vi "19.6-DirectIIR-SinglePole-HP.vi"() -> ()   [LabVIEW 2020]
doc: "Uses the Median Filter VI to analyze pulses in the presence of noise. The example generates a pulse contaminated with Gaussian noise and applies a median filter. For comparison purposes, the VI computes the pulse parameters of the filtered pulse."
uses:
  <vilib>/Analysis/3filter.llb/IIR Filter (DBL).vi
  <vilib>/Analysis/NI_AALBase.lvlib
panel:
  in  "stop":bool
  out "H[k] 2":dbl[](graph)
  out "Filtered2":dbl[](graph)
  out "Filtered1":dbl[](graph)
  out "H[k]1":dbl[](graph)
  out "p":dbl format="%.2f"
  in  "Fc":dbl(slide)=25.974025974025974 scale=0.0..400.0
  in  "Fs":dbl(slide)=1024.0 scale=800.0..1024.0
  out "Sig":dbl[](graph)
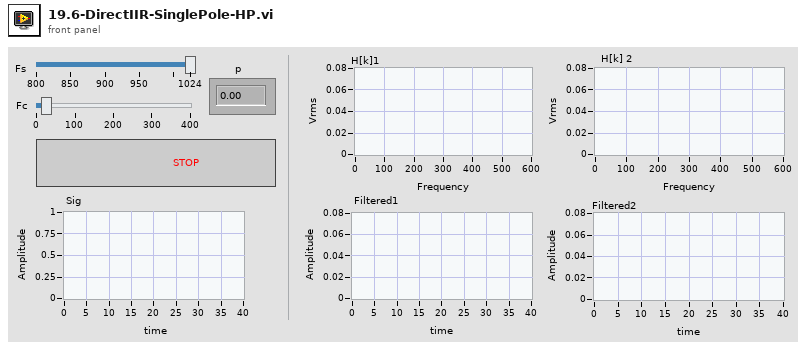
[diagram p1: front panel]
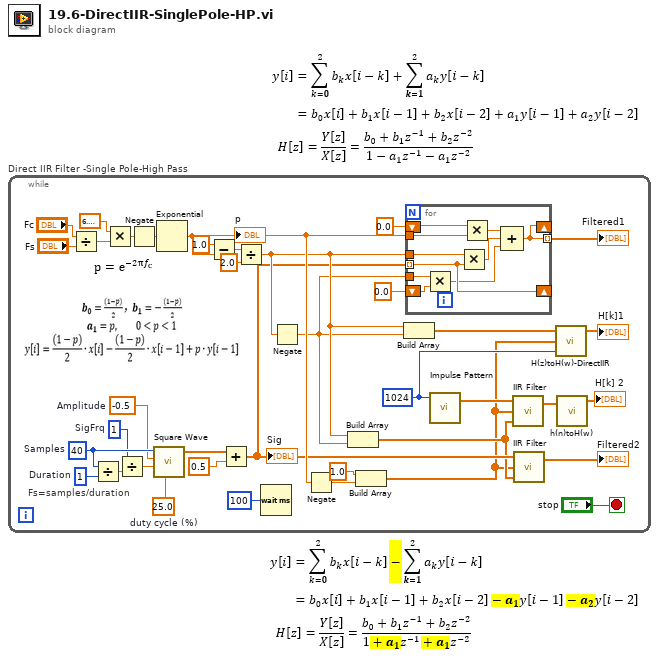
[diagram p0: block diagram]
diagram:
  n1 = while "Direct IIR Filter -Single Pole-High Pass" {
    stop <- "stop" stop-if-true
    w11 = 1  # Duration
    w8 = 1  # SigFrq
    w6 = 25.0  # duty cycle (%)
    w7 = -0.5  # Amplitude
    w10 = 40  # Samples
    w2 = 1024 ("samples")
    # "Fs=samples/duration"
    n2 = Divide(x="Fc", y="Fs") -> (x/y=w27:dbl)
    n3 = Divide(x=w10, y=w11) -> (x/y=w21:dbl)
    n4 = Multiply(x=6.283185307179586, y=w27) -> (x*y=w25:dbl)
    n5 = Divide(x=w8, y=w21) -> (x/y=w20:dbl)
    n6 = Negate(x=w25) -> (-x=w26:dbl)
    n7 = call <vilib>:"Square Wave.vi"("samples"=w10, "amplitude"=w7, "frequency"=w20, "duty cycle (%)"=w6) -> ("square wave"=w19:dbl[])  [unwired: 2 in, 2 out]
    n8 = Exponential(1:w26) -> (0:w31:dbl)
    "p" <- w31
    n9 = Subtract(x=1.0, y=w31) -> (x-y=w28:dbl)
    n10 = Add(x=w19, y=0.5) -> (x+y=w22:dbl[])
    "Sig" <- w22
    n11 = Divide(x=w28, y=2.0) -> (x/y=w30:dbl)
    n12 = Wait (ms)(milliseconds to wait=u32 100) -> ()  [unwired: 1 out]
    n13 = Negate(x=w30) -> (-x=w29:dbl)
    n14 = Negate(x=w31) -> (-x=w16:dbl)
    n15 = Build Array(w30, w29) -> (w17:dbl[])
    n16 = Build Array(1.0 ("element"), w16) -> (w1:dbl[])
    n17 = Build Array(w30, w29) -> (w15:dbl[])
    n18 = for {
      tunnel: w22 -> [w45] mode=indexing
      shift-right: [w39] -> _
      shift-left: 0.0 -> [w48]
      tunnel: w31 -> [w47]
      tunnel: w30 -> [w46]
      tunnel: [w39] -> w35 mode=indexing
      shift-right: [w45] -> _
      shift-left: 0.0 -> [w43]
      tunnel: w29 -> [w44]
      n19 = Multiply(x=w44, y=w43) -> (x*y=w40:dbl)
      n20 = Multiply(x=w46, y=w45) -> (x*y=w41:dbl)
      n21 = Multiply(x=w48, y=w47) -> (x*y=w42:dbl)
      n22 = Compound Arithmetic op=ADD(w42, w41, w40) -> (w39:dbl)
    }
    "Filtered1" <- w35
    n23 = call <vilib>:"Impulse Pattern.vi"("samples"=w2) -> ("Impulse Pattern"=w18:dbl[])  [unwired: 2 in, 1 out]
    n24 = call-poly <vilib>:"IIR Filter.vi"("Forward Coefficients"=w17, "Reverse Coefficients"=w1, "X"=w18) -> ("Filtered X"=w32:dbl[])  [unwired: 1 in, 1 out]
    n25 = call-poly <vilib>:"IIR Filter.vi"("Forward Coefficients"=w17, "Reverse Coefficients"=w1, "X"=w22) -> ("Filtered X"=→"Filtered2":dbl[])  [unwired: 1 in, 1 out]
    n26 = call "H(z)toH(w)-DirectIIR.vi"("FFT size"=w2, "Reverse"=w1, "Forward"=w15) -> ("Mag H(w)"=→"H[k]1":dbl[])  [unwired: 2 out]
    n27 = call "h(n)toH(w).vi"("h(n)"=w32) -> ("Mag H(w)"=→"H[k] 2":dbl[])  [unwired: 1 in, 2 out]
  }
